vi "Remove Item by name.vi"(8 "error in (no error)":errorcluster, 10 "name":string, 11 "JSON Value In":refnum<class "JSON Value.lvclass">) -> (0 "error out":errorcluster, 2 "removed":bool, 3 "JSON Value Out":refnum<class "JSON Value.lvclass">)   [LabVIEW 2020, in "Library Commun.lvlib" / "JSON Value.lvclass"]
doc: "Removes a <b>JSON Value</b> in a JSON collection by <b>name</b>.\n\nCopyright 2012 James David Powell, Shaun Rumbell and Ton Plomp\nMore information on http://lavag.org/topic/16217-cr-json-labview"
uses:
  JSON Value.lvclass
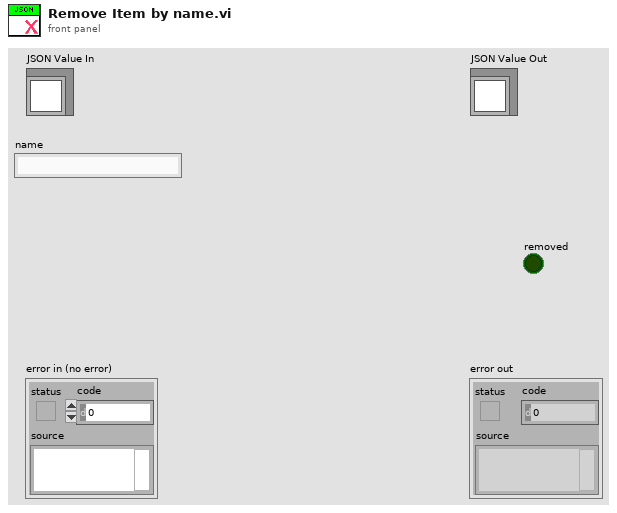
[diagram p1: front panel]
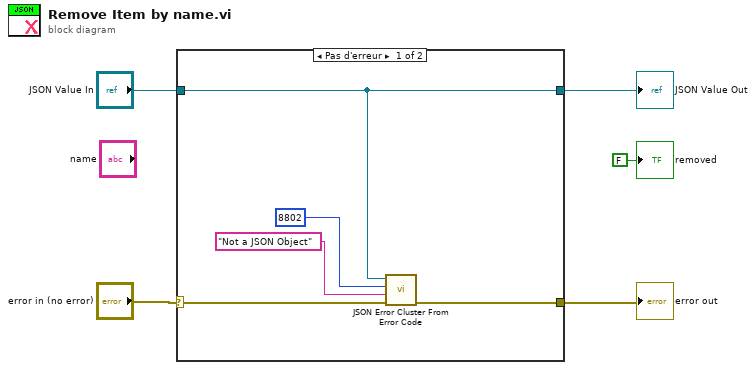
[diagram p0: block diagram]
diagram:
  n1 = case shown="Pas d'erreur" "error in (no error)" {
    selector: "error in (no error)" -> [w8 w12]
    tunnel: [w9 w12] -> w4
    tunnel: [w10 w11] -> w3
    tunnel: "JSON Value In" -> [w10 w11]
    frame No Error {
      n2 = call "JSON Error Cluster From Error Code.vi"("error in (no error)"=w8, "Error message"="Not a JSON Object", "JSON error code"=8802, "JSON Value in"=w10) -> ("error out"=w9:errorcluster)  [unwired: 6 in, 1 out]
    }
    frame Error {
    }
  }
  "error out" <- w4
  "JSON Value Out" <- w3
  "removed" <- FALSE ("found")
